vi "ep_Check Channel Number.vi"(0 "channel number":i32, 11 "error in (no error)":errorcluster) -> (15 "error out":errorcluster)   [LabVIEW 2014, in "NI_EP_Power Quality.lvlib"]
uses:
  <vilib>/addons/Electrical Power/PQ/NI_EP_Power Quality.lvlib
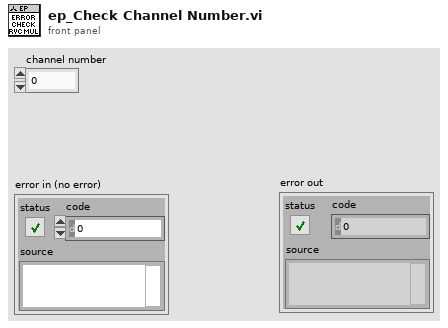
[diagram p1: front panel]
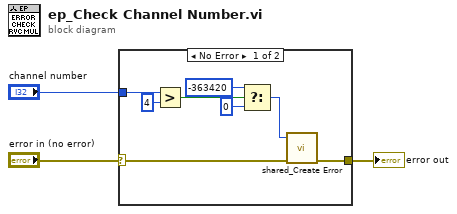
[diagram p0: block diagram]
diagram:
  n1 = case shown="No Error" "error in (no error)" {
    selector: "error in (no error)" -> [w5 w12]
    tunnel: [w4 w12] -> w2
    tunnel: "channel number" -> [w7 _]
    frame No Error {
      n2 = Greater?(x=w7, y=4 ("x")) -> (0:w10:bool)
      n3 = Select(t=-363420 ("error code (0)"), s=w10, f=0) -> (s? t:f=w8:i32)
      n4 = call <vilib>:"shared_Create Error.vi"("error in (no error)"=w5, "error code (0)"=w8) -> ("error out"=w4:errorcluster)  [unwired: 9 in]
    }
    frame Error {
    }
  }
  "error out" <- w2
